vi "Strategy 5_Autotuning PID_With GUI - Copy.vi"() -> ()   [LabVIEW 2018]
doc: "This example demonstrates how to use the PID Design function to obtain PID parameters based on measured process."
uses:
  <vilib>/DAQmx/write.llb/DAQmx Write (Digital 1D Bool 1Chan 1Samp).vi
  <vilib>/Instr/_visa.llb/VISA Configure Serial Port (Instr).vi
  <vilib>/DAQmx/create/channels.llb/DAQmx Create Channel (DO-Digital Output).vi
  <vilib>/DAQmx/miscellaneous.llb/DAQmx Fill In Error Info.vi
  <vilib>/addons/control/pid/pid.llb/PID Advanced (DBL).vi
  <vilib>/addons/control/pid/autopid.llb/PID Autotuning Design (Ziegler-Nichols).vi
  <vilib>/addons/control/pid/autopid.llb/PID Autotuning Design (Cohen-Coon).vi
  <vilib>/addons/control/pid/autopid.llb/PID Autotuning Design (Chien-Hrones-Reswick).vi
  <vilib>/addons/control/pid/autopid.llb/PID Autotuning Design (Internal Model Control).vi
  <vilib>/addons/control/pid/NI_PID_autopid.lvlib
  <vilib>/addons/control/pid/NI_PID_pid.lvlib
  <vilib>/ptbypt/NI_PtbyPt.lvlib
panel:
  out "?":bool
  in  "Muscle Control":T1(tab)=enum."M-11"
  in  "INLET":bool=TRUE
  out "PWM Output":bool
  out "Real time Data":dbl[][](graph)
  in  "MV:":dbl(slide)=20.39115328927357 scale=-100.0..100.0
  in  "Set Point":dbl(slide) scale=0.0..30.0
  in  "Median sample length":i32=100
  in  "Excitation":dbl=0.5 format="%.2f"
  in  "Type of controller":u16(ring)=2 items=["P", "PI", "PID"]
  in  "Control":T2(tab)
  in  "Ziegler-Nichols speed":u16(ring) items=["Fast", "Normal", "Slow"]
  in  "Tuning specifications":u16(ring) items=["Regulator - 0 %", "Regulator -  20%", "Servo - 0%", "Servo - 20%"]
  in  "Multiplicative factor":dbl(slide)=1.0 scale=0.01..100.0
  in  "Automatic":bool=TRUE
  in  "Reinitialize":bool
  in  "Accept gain":bool
  out "Tuned PID gains":T3={"proportional gain (Kc)"=1.9838195929127882, "integral time (Ti, min)"=0.01995856284686879, "derivative time (Td, min)"=0.0} {"derivative time (Td, min)" format="%#.6g"; "integral time (Ti, min)" format="%#.6g"; "proportional gain (Kc)" format="%#.6g"}
  in  "Autotune":bool
  in  "PID Gains":T3={"proportional gain (Kc)"=0.1625, "integral time (Ti, min)"=1.25, "derivative time (Td, min)"=0.0} {"derivative time (Td, min)" format="%#.6g"; "integral time (Ti, min)" format="%#.6g"; "proportional gain (Kc)" format="%#.6g"}
  in  "Stop":bool
  in  "M-11":i32=5
  out "Identified Plant Parameters":T4={"Plant Gain (K)"=1.7609511324977591, "Time Constant (T)"=1.9621978490901302, "Dead Time (L)"=0.22467425343567116}
  out "Control Output":dbl[](graph)
  out "Measurement":dbl[](graph)
  out "Stimulus operating point":dbl=20.314221540357543
  out "Response operating point":dbl=51.08345461694337
  in  "XYZAER":T5(array[cluster]) {"r" format="%1_6f"; "e" format="%1_6f"; "a" format="%1_6f"; "z" format="%1_6f"; "y" format="%1_6f"; "x" format="%1_6f"}
  out "Connected":bool
  out "Start Time Text":string
  out "Stop Time Text":string
  out "Elapsed Time Text":string
  out "HostFrameCount":u32
  out "Running":bool
  out "Loop Iter":i32
  out "PnoData":bool
  in  "stop":bool
  out "error out":errorcluster {"code" format="%.0x"}
  out "Position Sensor Data":cluster{dbl, "x":sgl}[](graph)
  out "Sensor Raw Value 2":i32
  in  "COM Port-Sensor 2":refnum<visa-resource-name>="COM5"
  in  "upper/lower infle":enum32{"Page 1", "Page 2"}(tab)
  out "Force in Kilograms":dbl(graph)
  out "Force in Newtons":dbl(graph)
  in  "lower/upper infle":enum32{"Page 1", "Page 2"}(tab)
  out "Force in Newtons 2":dbl(graph)
  out "Force in Kilograms 2":dbl(graph)
  in  "COM Port-Sensor 1":refnum<visa-resource-name>="COM4"
  out "Sensor Raw Value":i32
  in  "Tab Control":T6(tab)
  in  "Instructions":string="Overview: This example demonstrates how to use the PID Autotuning Design to obtain PID parameters based on setpoint and process variable collected in another loop.\nInstructions:\n1. Run the VI and wait until the process variable (PV) reaches near setpoint (SP).\n2.  In the PID Autotuning Design section, select the type of algorithm, type of controller and excitation amplitude for the 'open loop step response'. Then, click Autotune to start the process. Select the Identified Plant Parameter tab and see the results from the identification.\n3.  When the tuned PID gains do not change anymore, the identification is done and you have the option to accept by clicking Accept gain, which will transfer the new gain to PID Gains.\n4. Click the Autotune button again to go back to the automatic control state. You can try different options and repeat this process.\n5. Click Stop to stop the VI.\n"
  in  "Instructions 2":string="Overview: This example demonstrates how to use the PID Autotuning Design to obtain PID parameters based on setpoint and process variable collected in another loop.\nInstructions:\n1. Run the VI and wait until the process variable (PV) reaches near setpoint (SP).\n2.  In the PID Autotuning Design section, select the type of algorithm, type of controller and excitation amplitude for the 'open loop step response'. Then, click Autotune to start the process. Select the Identified Plant Parameter tab and see the results from the identification.\n3.  When the tuned PID gains do not change anymore, the identification is done and you have the option to accept by clicking Accept gain, which will transfer the new gain to PID Gains.\n4. Click the Autotune button again to go back to the automatic control state. You can try different options and repeat this process.\n5. Click Stop to stop the VI.\n"
  in  "Instructions 3":string="Overview: This example demonstrates how to use the PID Autotuning Design to obtain PID parameters based on setpoint and process variable collected in another loop.\nInstructions:\n1. Run the VI and wait until the process variable (PV) reaches near setpoint (SP).\n2.  In the PID Autotuning Design section, select the type of algorithm, type of controller and excitation amplitude for the 'open loop step response'. Then, click Autotune to start the process. Select the Identified Plant Parameter tab and see the results from the identification.\n3.  When the tuned PID gains do not change anymore, the identification is done and you have the option to accept by clicking Accept gain, which will transfer the new gain to PID Gains.\n4. Click the Autotune button again to go back to the automatic control state. You can try different options and repeat this process.\n5. Click Stop to stop the VI.\n"
  # "Pressure Alarm"
  # "Position Sensor Data"
  # "Force Sensor Data"
  # "Muscle Control"
  # "Muscle Control"
  # "PID Controller"
  # "PID Autotuning Design"
  # "No additional parameters"
  # "Pressure Cut Off to trigger the alarm"
  # "M-11"
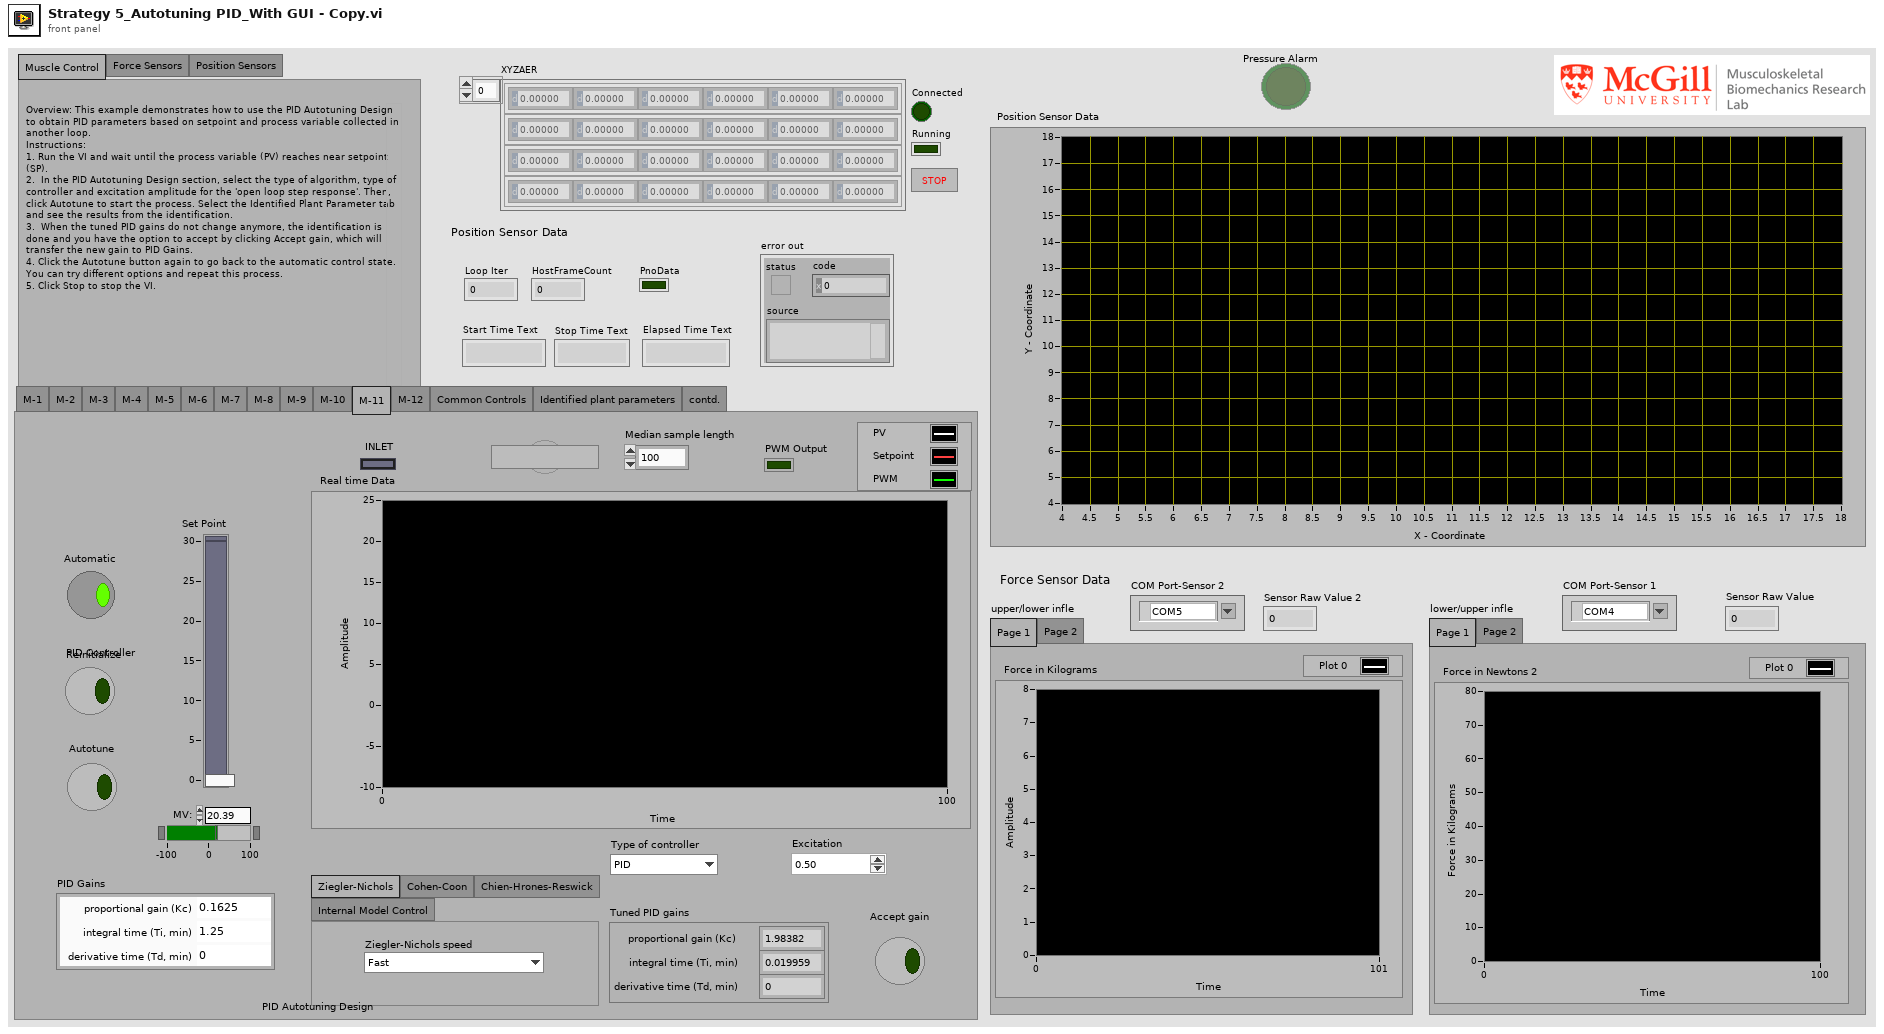
[diagram p1: front panel]
types:
  T1 = enum32{"M-1", "M-2", "M-3", "M-4", "M-5", "M-6", "M-7", "M-8", "M-9", "M-10", "M-11", "M-12", "Common Controls", "Identified plant parameters", "contd."}
  T2 = enum32{"Ziegler-Nichols", "Cohen-Coon", "Chien-Hrones-Reswick", "Internal Model Control"}
  T3 = cluster{"proportional gain (Kc)":dbl, "integral time (Ti, min)":dbl, "derivative time (Td, min)":dbl}
  T4 = cluster{"Plant Gain (K)":dbl, "Time Constant (T)":dbl, "Dead Time (L)":dbl}
  T5 = cluster{"x":sgl, "y":sgl, "z":sgl, "a":sgl, "e":sgl, "r":sgl}[]
  T6 = enum32{"Muscle Control", "Force Sensors", "Position Sensors"}
  T7 = cluster{"static gain":dbl, "lag (s)":dbl, "deadtime (s)":dbl, "load":dbl, "deadband":dbl, "sensor noise":dbl, "initial PV":dbl, "plant noise":dbl}
  T8 = cluster{"x":sgl, "y":sgl, "z":sgl, "a":sgl, "e":sgl, "r":sgl}
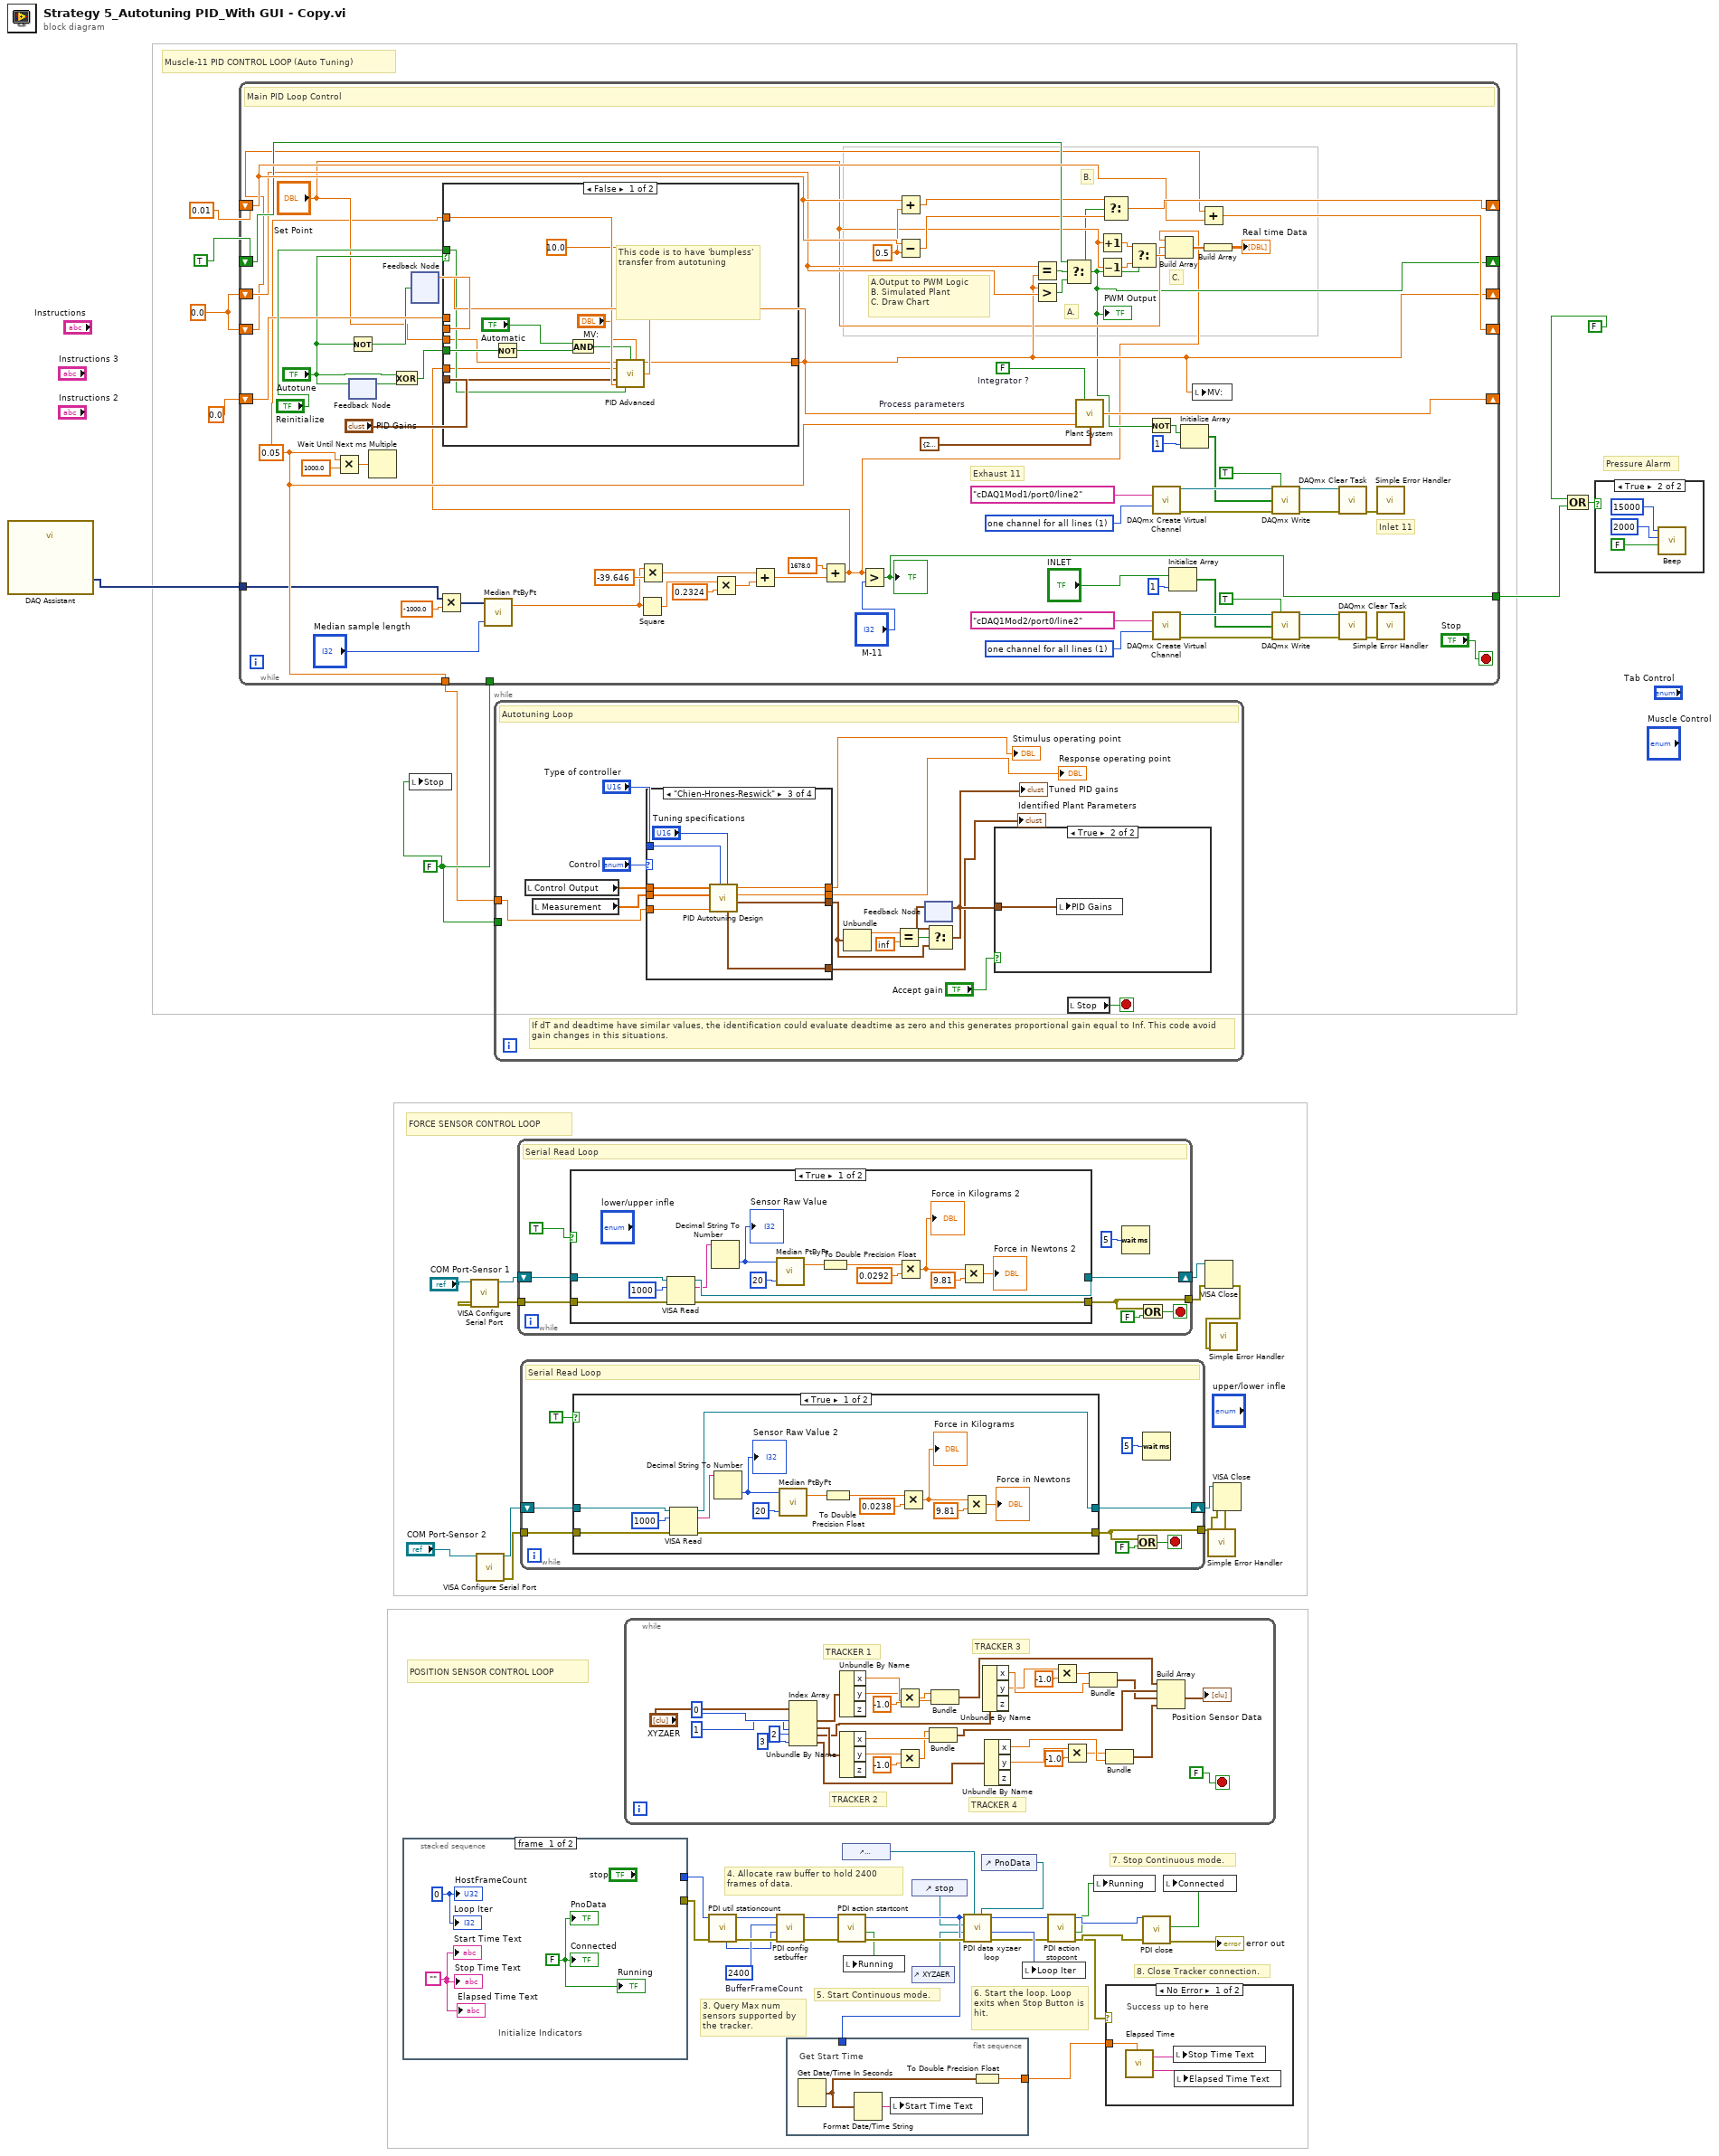
[diagram p0: block diagram]
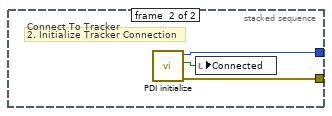
[diagram p4: hidden frame]
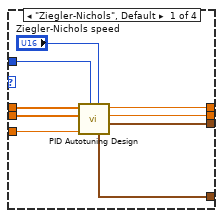
[diagram p7: hidden frame]
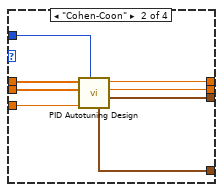
[diagram p8: hidden frame]
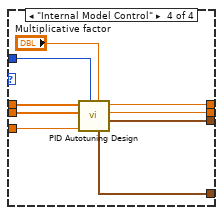
[diagram p9: hidden frame]
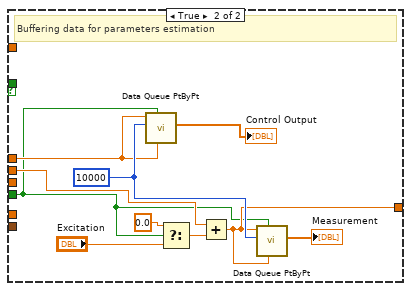
[diagram p11: hidden frame]
diagram:
  w8 = 2400  # BufferFrameCount
  w42 = 0.0 ("output")
  w45 = FALSE ("Stop")
  # "Muscle-11 PID CONTROL LOOP (Auto Tuning)"
  # "FORCE SENSOR CONTROL LOOP"
  # "POSITION SENSOR CONTROL LOOP"
  # "Pressure Alarm"
  # "8. Close Tracker connection."
  # "3. Query Max num sensors supported by the tracker."
  # "4. Allocate raw buffer to hold 2400 frames of data."
  # "5. Start Continuous mode."
  # "7. Stop Continuous mode."
  # "6. Start the loop. Loop exits when Stop Button is hit."
  n1 = call "DAQ Assistant"() -> ("data"=w4:dynamicdata)  [unwired: 17 in, 2 out]
  n2 = while {
    shift-left: 0.0 ("Plant Output") -> [w112]
    shift-right: [w107] -> _
    tunnel: w45 -> [_]
    shift-right: [w93] -> _
    shift-left: 0.01 -> [w91]
    shift-right: [w65] -> _
    shift-left: TRUE -> [w90]
    shift-right: [w67] -> _
    shift-left: w42 -> [w89]
    shift-right: [w92] -> _
    shift-left: w42 -> [w88]
    tunnel: [w62] -> w41
    tunnel: [w59] -> w3
    tunnel: w4 -> [w47]
    stop <- "Stop" stop-if-true
    w52 = 1 items=["one channel for each line", "one channel for all lines"] ("line grouping")
    w62 = 0.05 ("Sampling Time dt (s)")
    w71 = 1 items=["one channel for each line", "one channel for all lines"] ("line grouping")
    w79 = 0.5 ("x")
    w106 = T7 {"static gain"=2.5, "lag (s)"=2.5, "deadtime (s)"=0.01, "load"=0.0, "deadband"=0.0, "sensor noise"=0.0, "initial PV"=30.0, "plant noise"=0.0}  # Process parameters
    w108 = FALSE  # Integrator ?
    # "C."
    # "Inlet 11"
    # "Exhaust 11"
    # "B."
    # "A."
    # "A.Output to PWM Logic \nB. Simulated Plant\nC. Draw Chart"
    # "Main PID Loop Control"
    n3 = Multiply(x=w62, y=1000.0) -> (x*y=w105:dbl)
    n4 = Not(x="Autotune") -> (.not. x?=w109:bool)
    n5 = feedback #1() -> (w114:bool)  [unwired: 1 in]
    n6 = feedback-in #1("Autotune") -> ()
    n7 = Wait Until Next ms Multiple(millisecond multiple=w105) -> ()  [unwired: 1 out]
    n8 = Exclusive Or(1:w114, 2:"Autotune") -> (0:w113:bool)
    n9 = feedback #2() -> (w111:dbl)  [unwired: 1 in]
    n10 = Multiply(x=w47, y=-1000.0) -> (x*y=w95:dynamicdata)
    n11 = call <vilib>:"Median PtByPt.vi"("sample length"="Median sample length", "x"=w95) -> ("median"=w94:dbl)  [unwired: 2 in, 1 out]
    n12 = Square(x=w94) -> (x^2=w102:dbl)
    n13 = Multiply(x=w94, y=-39.646) -> (x*y=w98:dbl)
    n14 = Multiply(x=w102, y=0.2324) -> (x*y=w99:dbl)
    n15 = Add(x=w98, y=w99) -> (x+y=w97:dbl)
    n16 = Add(x=1678.0, y=w97) -> (x+y=w60:dbl)
    n17 = case shown="False" "Autotune" {
      tunnel: w62 -> [w129 _]
      tunnel: [w118 w134] -> w67
      tunnel: w112 -> [_ w133]
      tunnel: "PID Gains" -> [w128 _]
      tunnel: "Reinitialize" -> [w125 _]
      tunnel: w113 -> [w127 w132]
      tunnel: w111 -> [_ w136]
      tunnel: w60 -> [w121 _]
      tunnel: "Set Point" -> [w120 _]
      frame False {
        # "This code is to have 'bumpless' transfer from autotuning"
        n18 = Not(x=w127) -> (.not. x?=w124:bool)
        n19 = And(x="Automatic", y=w124) -> (x .and. y?=w126:bool)
        n20 = call-poly <vilib>:"PID Advanced.vi"("setpoint"=w120, "auto? (T)"=w126, "manual control"="MV:", "process variable"=w121, "alpha"=10.0, "PID gains"=w128, "dt (s)"=w129, "reinitialize? (F)"=w125) -> ("output"=w118:dbl)  [unwired: 6 in, 1 out]
      }
      frame True {
        w139 = 10000 ("sample length")
        # "Buffering data for parameters estimation"
        n21 = call <vilib>:"Data Queue PtByPt.vi"("initial queue element"=w133, "initialize"=w132, "sample length"=w139, "input data point"=w133) -> ("Current Queue"=→"Control Output":dbl[])  [unwired: 3 in, 4 out]
        n22 = Select(t=0.0, s=w132, f="Excitation") -> (s? t:f=w137:dbl)
        n23 = Add(x=w136, y=w137) -> (x+y=w134:dbl)
        n24 = call <vilib>:"Data Queue PtByPt.vi"("initial queue element"=w134, "initialize"=w132, "sample length"=w139, "input data point"=w134) -> ("Current Queue"=→"Measurement":dbl[])  [unwired: 3 in, 4 out]
      }
    }
    n25 = feedback-in #2(w67, w109) -> ()
    n26 = Greater?(x=w60, y="M-11") -> (0:w59:bool)
    "?" <- w59
    n27 = Add(x=w91, y=w79) -> (x+y=w80:dbl)
    n28 = Subtract(x=w91, y=w79) -> (x-y=w78:dbl)
    n29 = Equal?(x=w89, y=w67) -> (x = y?=w86:bool)
    n30 = Greater?(x=w67, y=w89) -> (0:w85:bool)
    n31 = Select(t=w90, s=w86, f=w85) -> (s? t:f=w65:bool)
    "PWM Output" <- w65
    n32 = call "Plant System.vi"("Integrator ?"=w108, "Plant Input"=w67, "dt (s)"=w62, "process parameters"=w106) -> ("Plant Output"=w107:dbl)  [unwired: 11 in]
    n33 = Increment(x="Set Point") -> (x+1=w84:dbl)
    n34 = Decrement(x="Set Point") -> (x-1=w83:dbl)
    n35 = Select(t=w80, s=w65, f=w78) -> (s? t:f=w93:dbl)
    n36 = Select(t=w84, s=w65, f=w83) -> (s? t:f=w82:dbl)
    n37 = Not(x=w65) -> (.not. x?=w64:bool)
    n38 = call-poly <vilib>:"DAQmx Create Virtual Channel.vi"("lines"=tag "cDAQ1Mod1/port0/line2", "line grouping"=w71) -> ("task out"=w73:refnum<k21>, "error out"=w72:errorcluster)  [unwired: 12 in]
    n39 = call-poly <vilib>:"DAQmx Create Virtual Channel.vi"("lines"=tag "cDAQ1Mod2/port0/line2", "line grouping"=w52) -> ("task out"=w54:refnum<k21>, "error out"=w53:errorcluster)  [unwired: 12 in]
    n40 = Build Array(w60, "Set Point", w82) -> (w81:dbl[])
    n41 = Initialize Array("INLET", 1 ("dimension size")) -> (w49:bool[])
    n42 = Initialize Array(w64, 1 ("dimension size")) -> (w68:bool[])
    n43 = local write "MV:"(w67) -> ()
    n44 = Add(x=w88, y=w91) -> (x+y=w92:dbl)
    n45 = Build Array(w81) -> (→"Real time Data":dbl[][])
    n46 = call-poly <vilib>:"DAQmx Write.vi"("task/channels in"=w73, "auto start"=TRUE, "data"=w68, "error in"=w72) -> ("task out"=w75:refnum<k21>, "error out"=w76:errorcluster)  [unwired: 9 in, 1 out]
    n47 = call-poly <vilib>:"DAQmx Write.vi"("task/channels in"=w54, "auto start"=TRUE, "data"=w49, "error in"=w53) -> ("task out"=w56:refnum<k21>, "error out"=w57:errorcluster)  [unwired: 9 in, 1 out]
    n48 = call <vilib>:"DAQmx Clear Task.vi"("task in"=w75, "error in"=w76) -> ("error out"=w70:errorcluster)  [unwired: 13 in]
    n49 = call <vilib>:"DAQmx Clear Task.vi"("task in"=w56, "error in"=w57) -> ("error out"=w51:errorcluster)  [unwired: 13 in]
    n50 = call <vilib>:"Simple Error Handler.vi"("error in (no error)"=w70) -> ()  [unwired: 4 in, 5 out]
    n51 = call <vilib>:"Simple Error Handler.vi"("error in (no error)"=w51) -> ()  [unwired: 4 in, 5 out]
  }
  n52 = stacked-sequence {
    tunnel: [_ w145] -> w12
    tunnel: [_ w144] -> w11
    frame #0 {
      w140 = 0
      w141 = FALSE
      w142 = ""
      # "Initialize Indicators"
      "Connected" <- w141
      "Start Time Text" <- w142
      "Stop Time Text" <- w142
      "Elapsed Time Text" <- w142
      "HostFrameCount" <- w140
      "Running" <- w141
      "Loop Iter" <- w140
      "PnoData" <- w141
    }
    frame #1 {
      # "Connect To Tracker"
      # "2. Initialize Tracker Connection"
      n53 = call <instrlib>:"PDI initialize.vi"() -> ("error out"=w144:errorcluster, "Connected"=w143:bool, "pDev"=w145:u32)  [unwired: 1 in, 4 out]
      n54 = local write "Connected"(w143) -> ()
    }
  }
  n55 = local write "Stop"(w45) -> ()
  n56 = call-poly "VISA Configure Serial Port"("VISA resource name"="COM Port-Sensor 1") -> ("VISA resource name out"=w36:refnum<visa-resource-name>, "error out"=w35:errorcluster)  [unwired: 9 in, 4 out]
  n57 = call-poly "VISA Configure Serial Port"("VISA resource name"="COM Port-Sensor 2") -> ("VISA resource name out"=w31:refnum<visa-resource-name>, "error out"=w30:errorcluster)  [unwired: 9 in, 4 out]
  n58 = while {
    tunnel: w45 -> [_]
    tunnel: w41 -> [w149]
    stop <- w159 stop-if-true
    # "If dT and deadtime have similar values, the identification could evaluate deadtime as zero and this generates proportional gain equal to Inf. This code avoid gain changes in this situations."
    # "Autotuning Loop"
    n59 = local read "Control Output"() -> (w161:dbl[])
    n60 = local read "Measurement"() -> (w160:dbl[])
    n61 = case shown="\"Chien-Hrones-Reswick\"" "Control" {
      tunnel: w161 -> [w170 w178 w187 w196]
      tunnel: w160 -> [w169 w177 w186 w195]
      tunnel: [w168 w176 w185 w194] -> w148
      tunnel: [w167 w175 w184 w193] -> w147
      tunnel: w149 -> [w166 w174 w183 w192]
      tunnel: [w165 w173 w182 w191] -> w146
      tunnel: [w164 w172 w181 w190] -> w151
      tunnel: "Type of controller" -> [w163 w171 w180 w189]
      frame "Ziegler-Nichols", Default {
        n62 = call-poly <vilib>:"PID Autotuning Design.vi"("Ziegler-Nichols Speed"="Ziegler-Nichols speed", "Type of Controller"=w163, "dt (s)"=w166, "Response signal"=w169, "Stimulus signal"=w170) -> ("PID gains"=w164:T3, "response operating point"=w167:dbl, "stimulus operating point"=w168:dbl, "Plant Parameters"=w165:T4)  [unwired: 3 in]
      }
      frame "Cohen-Coon" {
        n63 = call-poly <vilib>:"PID Autotuning Design.vi"("Type of Controller"=w171, "dt (s)"=w174, "Response signal"=w177, "Stimulus signal"=w178) -> ("PID gains"=w172:T3, "response offset"=w175:dbl, "stimulus offset"=w176:dbl, "Plant Parameters"=w173:T4)  [unwired: 4 in]
      }
      frame "Chien-Hrones-Reswick" {
        n64 = call-poly <vilib>:"PID Autotuning Design.vi"("Tuning specifications"="Tuning specifications", "Type of Controller"=w180, "dt (s)"=w183, "Response signal"=w186, "Stimulus signal"=w187) -> ("PID gains"=w181:T3, "response offset"=w184:dbl, "stimulus offset"=w185:dbl, "Plant Parameters"=w182:T4)  [unwired: 3 in]
      }
      frame "Internal Model Control" {
        n65 = call-poly <vilib>:"PID Autotuning Design.vi"("Desired Time Constant (tau_c)"="Multiplicative factor", "Type of Controller"=w189, "dt (s)"=w192, "Response signal"=w195, "Stimulus signal"=w196) -> ("PID gains"=w190:T3, "response offset"=w193:dbl, "stimulus offset"=w194:dbl, "Plant Parameters"=w191:T4)  [unwired: 3 in]
      }
    }
    "Stimulus operating point" <- w148
    "Response operating point" <- w147
    "Identified Plant Parameters" <- w146
    n66 = Unbundle(w151) -> ("proportional gain (Kc)"=w154:dbl)  [unwired: 2 out]
    n67 = Equal?(x=w154, y=inf) -> (x = y?=w153:bool)
    n68 = feedback #3() -> (w152:T3)  [unwired: 1 in]
    n69 = Select(t=w152, s=w153, f=w151) -> (s? t:f=w150:T3)
    "Tuned PID gains" <- w150
    n70 = feedback-in #3(w150) -> ()
    n71 = case shown="True" "Accept gain" {
      tunnel: w150 -> [_ w197]
      frame False {
      }
      frame True {
        n72 = local write "PID Gains"(w197) -> ()
      }
    }
    n73 = local read "Stop"() -> (w159:bool)
  }
  n74 = while {
    shift-right: [w205] -> w37
    shift-left: w36 -> [w201]
    tunnel: w35 -> [w200]
    tunnel: [w202] -> w38
    stop <- w203 stop-if-true
    # "Serial Read Loop"
    n75 = case shown="True" TRUE {
      tunnel: [w217 w221] -> w205
      tunnel: w201 -> [w219 w221]
      tunnel: [w216 w220] -> w202
      tunnel: w200 -> [w218 w220]
      frame True {
        n76 = VISA Read(VISA resource name=w219, byte count=u32 1000, error in (no error)=w218) -> (VISA resource name out=w217:refnum<visa-resource-name>, read buffer=w214:string, error out=w216:errorcluster)  [unwired: 1 out]
        n77 = Decimal String To Number(string=w214) -> (number=w212:i32)  [unwired: 2 in, 1 out]
        "Sensor Raw Value" <- w212
        n78 = call <vilib>:"Median PtByPt.vi"("sample length"=20, "x"=w212) -> ("median"=w210:dbl)  [unwired: 2 in, 1 out]
        n79 = To Double Precision Float(number=w210) -> (double precision float=w206:dbl)
        n80 = Multiply(x=w206, y=0.0292) -> (x*y=w209:dbl)
        "Force in Kilograms 2" <- w209
        n81 = Multiply(x=w209, y=9.81) -> (x*y=→"Force in Newtons 2":dbl)
      }
      frame False {
      }
    }
    n82 = Wait (ms)(milliseconds to wait=u32 5) -> ()  [unwired: 1 out]
    n83 = Or(x=w202, y=FALSE) -> (x .or. y?=w203:bool)
  }
  n84 = while {
    shift-right: [w229] -> w5
    shift-left: w31 -> [w225]
    tunnel: w30 -> [w224]
    tunnel: [w226] -> w32
    stop <- w227 stop-if-true
    # "Serial Read Loop"
    n85 = case shown="True" TRUE {
      tunnel: [w241 w245] -> w229
      tunnel: w225 -> [w243 w245]
      tunnel: [w240 w244] -> w226
      tunnel: w224 -> [w242 w244]
      frame True {
        n86 = VISA Read(VISA resource name=w243, byte count=u32 1000, error in (no error)=w242) -> (VISA resource name out=w241:refnum<visa-resource-name>, read buffer=w238:string, error out=w240:errorcluster)  [unwired: 1 out]
        n87 = Decimal String To Number(string=w238) -> (number=w234:i32)  [unwired: 2 in, 1 out]
        "Sensor Raw Value 2" <- w234
        n88 = call <vilib>:"Median PtByPt.vi"("sample length"=20, "x"=w234) -> ("median"=w235:dbl)  [unwired: 2 in, 1 out]
        n89 = To Double Precision Float(number=w235) -> (double precision float=w231:dbl)
        n90 = Multiply(x=w231, y=0.0238) -> (x*y=w230:dbl)
        "Force in Kilograms" <- w230
        n91 = Multiply(x=w230, y=9.81) -> (x*y=→"Force in Newtons":dbl)
      }
      frame False {
      }
    }
    n92 = Or(x=w226, y=FALSE) -> (x .or. y?=w227:bool)
    n93 = Wait (ms)(milliseconds to wait=u32 5) -> ()  [unwired: 1 out]
  }
  n94 = while {
    stop <- FALSE stop-if-true
    # "TRACKER 4"
    # "TRACKER 3"
    # "TRACKER 2"
    # "TRACKER 1"
    n95 = Index Array(array="XYZAER", index #1=0 ("index"), index #2=1 ("index"), index #3=2 ("index"), index #4=3 ("index")) -> (element #1=w270:T8, element #2=w269:T8, element #3=w268:T8, element #4=w267:T8)
    n96 = Unbundle By Name(w270) -> ("x"=w257:sgl, "y"=w256:sgl)  [unwired: 1 out]
    n97 = Unbundle By Name(w269) -> ("x"=w254:sgl, "y"=w253:sgl)  [unwired: 1 out]
    n98 = Multiply(x=w256, y=sgl -1.0) -> (x*y=w255:sgl)
    n99 = Multiply(x=w253, y=-1.0) -> (x*y=w252:dbl)
    n100 = Bundle(w252, "x"=w254) -> (w265:cluster{dbl, "x":sgl})  [unwired: 1 in]
    n101 = Bundle(w255, "x"=w257) -> (w266:cluster{sgl, "x":sgl})  [unwired: 1 in]
    n102 = Unbundle By Name(w268) -> ("x"=w251:sgl, "y"=w250:sgl)  [unwired: 1 out]
    n103 = Unbundle By Name(w267) -> ("x"=w248:sgl, "y"=w247:sgl)  [unwired: 1 out]
    n104 = Multiply(x=w250, y=-1.0) -> (x*y=w249:dbl)
    n105 = Multiply(x=w247, y=-1.0) -> (x*y=w246:dbl)
    n106 = Bundle(w249, "x"=w251) -> (w264:cluster{dbl, "x":sgl})  [unwired: 1 in]
    n107 = Bundle(w246, "x"=w248) -> (w263:cluster{dbl, "x":sgl})  [unwired: 1 in]
    n108 = Build Array(w266, w265, w264, w263) -> (→"Position Sensor Data":cluster{dbl, "x":sgl}[])
  }
  n109 = call <instrlib>:"PDI util stationcount.vi"("error in (no error)"=w11, "pDev"=w12) -> ("error out"=w10:errorcluster, "dup pDev"=w9:u32, "MaxCount"=w7:i32)  [unwired: 7 out]
  n110 = call <instrlib>:"PDI config setbuffer.vi"("error in (no error)"=w10, "Max sensors"=w7, "FrameCount"=w8, "pDev"=w9) -> ("error out"=w19:errorcluster, "dup pDev"=w20:u32)  [unwired: 6 out]
  n111 = flat-sequence {
    tunnel: w25 -> [_]
    tunnel: [w277] -> w21
    frame #0 {
      # "Get Start Time"
      n112 = Get Date/Time In Seconds() -> (seconds since 1Jan1904=w278:timestamp)
      n113 = Format Date/Time String(seconds (now)=w278) -> (date/time string=w279:string)  [unwired: 2 out]
      n114 = local write "Start Time Text"(w279) -> ()
      n115 = To Double Precision Float(number=w278) -> (double precision float=w277:dbl)
    }
  }
  n116 = call <instrlib>:"PDI action startcont.vi"("error in (no error)"=w19, "pDev"=w20) -> ("error out"=w26:errorcluster, "Running"=w18:bool, "dup pDev"=w25:u32)  [unwired: 7 out]
  n117 = control-ref of="HostFrameCount"() -> (w16:refnum<vi>)
  n118 = local write "Running"(w18) -> ()
  n119 = control-ref of="stop"() -> (w24:refnum<vi>)
  n120 = control-ref of="XYZAER"() -> (w15:refnum<vi>)
  n121 = control-ref of="PnoData"() -> (w6:refnum<vi>)
  n122 = call <instrlib>:"PDI data xyzaer loop.vi"("Data Ready Refnum"=w6, "FrameCount Ctl Ref"=w16, "error in (no error)"=w26, "xyzaer array\nRefnum"=w15, "Stop Ctl Ref"=w24, "pDev"=w25) -> ("error out"=w13:errorcluster, "Loop Iter"=w17:i32, "dup pDev"=w14:u32)  [unwired: 3 out]
  n123 = local write "Loop Iter"(w17) -> ()
  n124 = call <instrlib>:"PDI action stopcont.vi"("error in (no error)"=w13, "pDev"=w14) -> ("error out"=w22:errorcluster, "Running"=w27:bool, "dup pDev"=w28:u32)  [unwired: 7 out]
  n125 = local write "Running"(w27) -> ()
  n126 = case shown="No Error" w13 {
    tunnel: w21 -> [w280 _]
    frame No Error {
      # "Success up to here"
      n127 = call "Elapsed Time"("Set Start Time (s)"=w280) -> ("Present Text"=w282:string, "Elapsed Time Text"=w281:string)  [unwired: 4 in, 13 out]
      n128 = local write "Stop Time Text"(w282) -> ()
      n129 = local write "Elapsed Time Text"(w281) -> ()
    }
    frame Error {
      # "Error somewhere;\nStop Time is irrelevant"
    }
  }
  n130 = call <instrlib>:"PDI close.vi"("error in (no error)"=w22, "pDev"=w28) -> ("error out"=→"error out":errorcluster, "connected"=w23:bool)  [unwired: 8 out]
  n131 = local write "Connected"(w23) -> ()
  n132 = VISA Close(VISA resource name=w37, error in (no error)=w38) -> (error out=w39:errorcluster)
  n133 = call <vilib>:"Simple Error Handler.vi"("error in (no error)"=w39) -> ()  [unwired: 1 in, 8 out]
  n134 = VISA Close(VISA resource name=w5, error in (no error)=w32) -> (error out=w33:errorcluster)
  n135 = call <vilib>:"Simple Error Handler.vi"("error in (no error)"=w33) -> ()  [unwired: 1 in, 8 out]
  n136 = Compound Arithmetic op=OR(FALSE, w3) -> (w2:bool)
  n137 = case shown="True" w2 {
    frame False {
    }
    frame True {
      n138 = call <vilib>:"Beep.vi"("use system alert? (T)"=FALSE, "duration (msec)"=u32 2000, "frequency (Hz)"=u32 15000) -> ()  [unwired: 9 in]
    }
  }
